vi "Get Logout Path.vi"(8 "error in (no error)":errorcluster, 11 "Authentication Provider in":refnum<class "Authentication Provider.lvclass">) -> (0 "error out":errorcluster, 2 "Logout Path":string, 3 "Authentication Provider out":refnum<class "Authentication Provider.lvclass">)   [LabVIEW 2020, in "HTTP Server.lvlib" / "Authentication Provider.lvclass"]
uses:
  Authentication Provider.lvclass
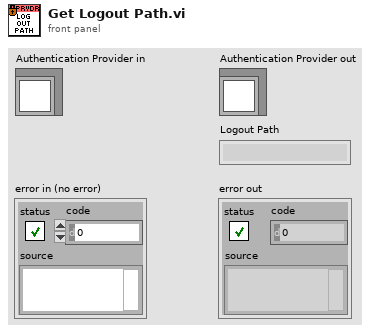
[diagram p1: front panel]
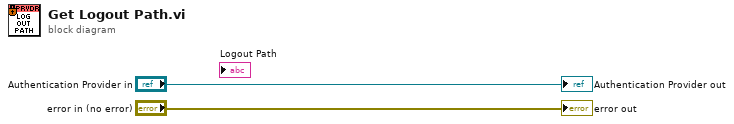
[diagram p0: block diagram]
diagram:
  "error out" <- "error in (no error)"
  "Authentication Provider out" <- "Authentication Provider in"
